vi "cmc_Time_Generator.vi"() -> ()   [LabVIEW 2010]
panel:
  in  "stop":bool
  out "Elapsed Time in ms":u32
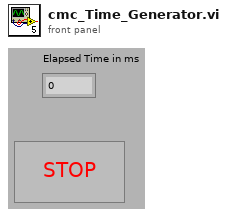
[diagram p1: front panel]
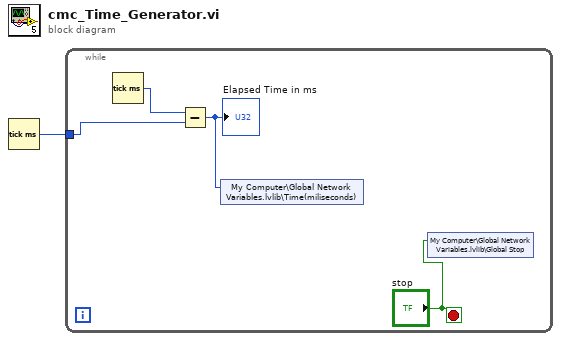
[diagram p0: block diagram]
diagram:
  n1 = Tick Count (ms)() -> (millisecond timer value=w1:u32)
  n2 = while {
    tunnel: w1 -> [w4]
    stop <- "stop" stop-if-true
    n3 = Tick Count (ms)() -> (millisecond timer value=w5:u32)
    n4 = Subtract(x=w5, y=w4) -> (x-y=w3:u32)
    "Elapsed Time in ms" <- w3
    n5 = shared-variable "My Computer\\Global Network Variables.lvlib\\Time(miliseconds)"(w3) -> ()  [unwired: 1 in, 1 out]
    n6 = shared-variable "My Computer\\Global Network Variables.lvlib\\Global Stop"("stop") -> ()  [unwired: 1 in, 1 out]
  }
